vi "VMI_create_arrays.vi"(9 "Collection Information":T1[](array[typedef]), 10 "Ysize":dbl, 11 "Xsize":dbl) -> (2 "Big_image Array":i16[][][](array[numeric]), 3 "Image Array":dbl[][](array[numeric]))   [LabVIEW 2020]
uses:
  Type defs/FileAcq_v1_Ctrl.ctl
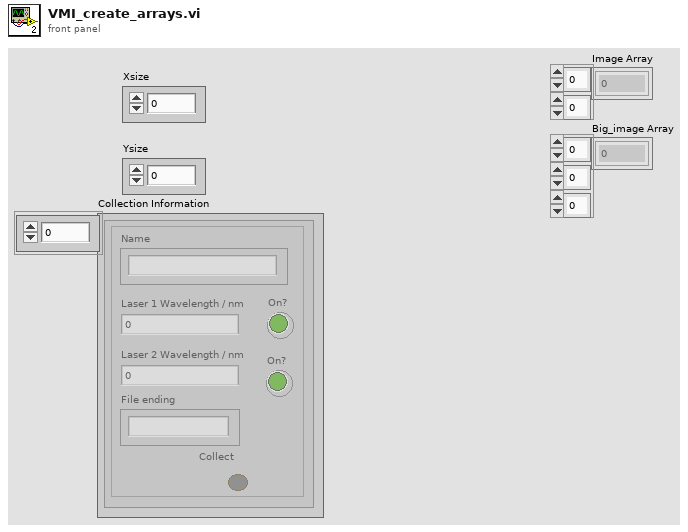
[diagram p1: front panel]
types:
  T1 = typedef "FileAcq_v1_Ctrl.ctl" = cluster{"Type":string, "LaserWave1":dbl, "Shutter1":bool, "LaserWave2":dbl, "Shutter2":bool, "FileEnd":string, "Collect":bool}
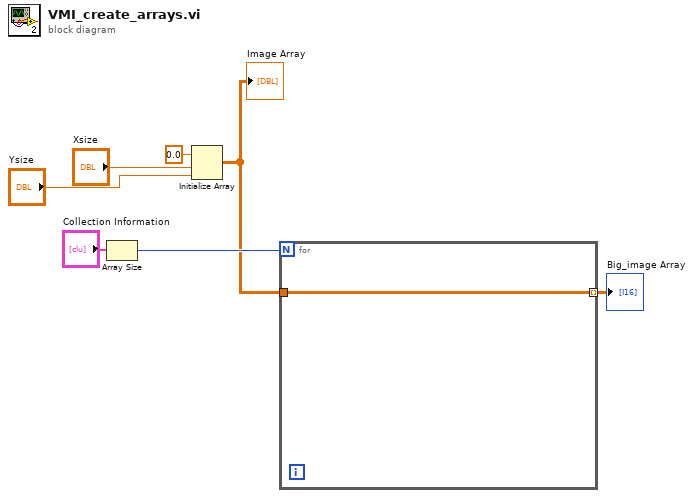
[diagram p0: block diagram]
diagram:
  n1 = Array Size(array="Collection Information") -> (size(s)=w3:i32)
  n2 = Initialize Array(0.0 ("element"), "Xsize", "Ysize") -> (w2:dbl[][])
  "Image Array" <- w2
  n3 = for {
    N: w3 -> [_]
    tunnel: w2 -> [w8]
    tunnel: [w8] -> w1 mode=indexing
  }
  "Big_image Array" <- w1
